vi "TektronixMDO_multiChannelReadout_writeFile.vi"(11 "file path":path=path "C:/Users/user01/Desktop/hsinyeh/SNSPD_Data/20230411/2.5M_6.1K_20photons_1.36uW_100mV") -> ()   [LabVIEW 2016]
doc: "This example illustrates how to use autosetup and continuously acquires waveforms from a single channel using the following steps:\n\n1. Specify a valid VISA session. \n2. Specify a channel. \n3. Specify a time-out value for reading waveform.\n4. Run the VI. The graph displays the waveform you acquire."
uses:
  <instrlib>/Tektronix DPO MSO 2000 4000 Series/Public/Configure/Configure Trigger (Edge).vi
  <instrlib>/Tektronix DPO MSO 2000 4000 Series/Public/Data/Read (Multiple Waveforms).vi
  <instrlib>/Tektronix DPO MSO 2000 4000 Series/Tektronix DPO MSO 2000 4000 Series.lvlib
panel:
  out "sum of values":dynamicdata(graph)=[{"t0"=timestamp(0.005 s since 1904-01-01), "dt"=0.01, "Y"=[0.0, 0.0, 0.0, 0.0, 0.0, 0.0, 0.0, 0.0, 0.0, 0.0, 0.0, 0.0, 0.0, 0.0, 0.0, 0.0, 0.0, 0.0, 0.0, 0.0, 0.0, 0.0, 0.0, 0.0, 0.0, 0.0, 0.0, 0.0, 0.0, 0.0, 0.0, 0.0, 0.0, 0.0, 0.0, 0.0, 0.0, 0.0, 0.0, 0.0, 0.0, 0.0, 0.0, 0.0, 0.0, 0.0, 0.0, 0.0, 0.0, 0.0], "attributes"=variant("NI_ChannelName"=variant(string "Summation (Histogram)"), "NI_ExpIsRelativeTime"=variant(bool TRUE), "NI_ExpStartTimeStamp"=variant(timestamp timestamp(0 s since 1904-01-01)), "NI_ExpTimeStamp"=variant(timestamp timestamp(0 s since 1904-01-01)), "NI_ExpXDimension"=variant(string "BIN"), "NI_OriginalChannelName"=variant(string "Summation"))}] caption="Histogram"
  in  "Enable Channel 3":bool
  in  "Vertical Coupling (1: DC) 3":u16(ring)=1 items=["AC", "DC", "Ground", "DC Reject"]
  in  "Probe Attenuation (1) 3":dbl=1.0
  in  "Vertical Offset (0.0 V) 3":dbl
  in  "Input Impedance 3":u16(ring) items=["1M", "75", "50"]
  in  "Vertical Range (10.0 V) 3":dbl=10.0
  in  "Bandwidth (0: FULL) 3":u16(ring) items=["FULL", "250 MHz", "150 MHz", "20 MHz"]
  in  "Enable Channel 4":bool
  in  "Input Impedance 4":u16(ring) items=["1M", "75", "50"]
  in  "Vertical Coupling (1: DC) 4":u16(ring)=1 items=["AC", "DC", "Ground", "DC Reject"]
  in  "Probe Attenuation (1) 4":dbl=1.0
  in  "Vertical Range (10.0 V) 4":dbl=10.0
  in  "Vertical Offset (0.0 V) 4":dbl
  in  "Bandwidth (0: FULL) 4":u16(ring) items=["FULL", "250 MHz", "150 MHz", "20 MHz"]
  in  "Enable Channel 2":bool=TRUE
  in  "Input Impedance 2":u16(ring)=2 items=["1M", "75", "50"]
  in  "Vertical Coupling (1: DC) 2":u16(ring)=1 items=["AC", "DC", "Ground", "DC Reject"]
  in  "Probe Attenuation (1) 2":dbl=1.0
  in  "Vertical Range (10.0 V) 2":dbl=1.0
  in  "Vertical Offset (0.0 V) 2":dbl
  in  "Bandwidth (0: FULL) 2":u16(ring) items=["FULL", "250 MHz", "150 MHz", "20 MHz"]
  in  "Input Impedance":u16(ring)=2 items=["1M", "75", "50"]
  in  "Vertical Coupling (1: DC)":u16(ring)=1 items=["AC", "DC", "Ground", "DC Reject"]
  in  "Vertical Range (10.0 V)":dbl=0.01
  in  "Vertical Offset (0.0 V)":dbl
  in  "Bandwidth (0: FULL)":u16(ring) items=["FULL", "250 MHz", "150 MHz", "20 MHz"]
  in  "Probe Attenuation (1)":dbl=1.0
  in  "Enable Channel":bool=TRUE
  in  "Trigger Source":u16(ring)=1 items=["Channel 1", "Channel 2", "Channel 3", "Channel 4", "AC Line", "Aux", "Digital Channel 0", "Digital Channel 1", "Digital Channel 2", "Digital Channel 3", "Digital Channel 4", "Digital Channel 5", "Digital Channel 6", "Digital Channel 7", "Digital Channel 8", "Digital Channel 9", "Digital Channel 10", "Digital Channel 11", "Digital Channel 12", "Digital Channel 13", "Digital Channel 14", "Digital Channel 15", "RF"]
  out "Event rate":dbl=1.5321756894790601
  in  "Maximum Time (10000ms)":u32=10000
  in  "Timebase (0.0005 s)":dbl=1e-08
  in  "Position (10 %)":dbl=10.0
  in  "Record Length":u32(ring)=10 items=["1000 points"=1, "10k points"=10, "100k points"=100, "1M points"=1000, "5M points"=5000, "10M points"=10000]
  out "Event Count":i32=75
  in  "Target total event":i32=1
  out "dt":dbl=4e-10 format="%#_13g"
  out "range":dynamicdata(graph)=[{"t0"=timestamp(0.00014999999999999996 s since 1904-01-01), "dt"=0.0003, "Y"=[0.0, 0.0, 0.0, 0.0, 0.0, 0.0, 0.0, 0.0, 0.0, 0.0, 0.0, 0.0, 0.0, 0.0, 0.0, 0.0, 0.0, 0.0, 0.0, 0.0, 0.0, 0.0, 0.0, 0.0, 0.0, 0.0, 0.0, 0.0, 0.0, 0.0, 0.0, 0.0, 0.0, 0.0, 0.0, 0.0, 0.0, 0.0, 0.0, 0.0, 0.0, 0.0, 0.0, 0.0, 0.0, 0.0, 0.0, 0.0, 0.0, 0.0, 0.0, 0.0, 0.0, 0.0, 0.0, 0.0, 0.0, 0.0, 0.0, 0.0, 0.0, 0.0, 0.0, 0.0, 0.0, 0.0, 0.0, 0.0, 0.0, 0.0, 0.0, 0.0, 0.0, 0.0, 0.0, 0.0, 0.0, 0.0, 0.0, 0.0, 0.0, 0.0, 0.0, 0.0, 0.0, 0.0, 0.0, 0.0, 0.0, 0.0, 0.0, 0.0, 0.0, 0.0, 0.0, 0.0, 0.0, 0.0, 0.0, 0.0], "attributes"=variant("NI_ChannelName"=variant(string "Range (Histogram)"), "NI_ExpIsRelativeTime"=variant(bool TRUE), "NI_ExpStartTimeStamp"=variant(timestamp timestamp(0 s since 1904-01-01)), "NI_ExpTimeStamp"=variant(timestamp timestamp(0 s since 1904-01-01)), "NI_ExpXDimension"=variant(string "BIN"), "NI_OriginalChannelName"=variant(string "Range"))}] caption="Histogram"
  in  "Operator":string="Hsin-Yeh"
  in  "Trigger Slope (0: Rising)":u16(ring)=1 items=["Rising", "Falling", "Either"]
  in  "Trigger Level (0.0 V)":dbl=-0.5
  in  "Trigger Coupling (0 : DC)":u16(ring) items=["DC", "HF Reject", "LF Reject", "Noise Reject", "AC"]
  out "Waveform Graph":waveform(dbl)[](graph)=[{"t0"=timestamp(-1.916400000023799e-06 s since 1904-01-01), "dt"=4e-10, "Y"=array[10000 elements]}, {"t0"=timestamp(-1.916400000023799e-06 s since 1904-01-01), "dt"=4e-10, "Y"=array[10000 elements]}]
  in  "stop":bool
  in  "VISA Resource Name":refnum<visa-resource-name>="USB0::0x0699::0x0408::C022314::INSTR"
  # "Channel 4"
  # "Channel 3"
  # "Channel 2"
  # "Channel 1"
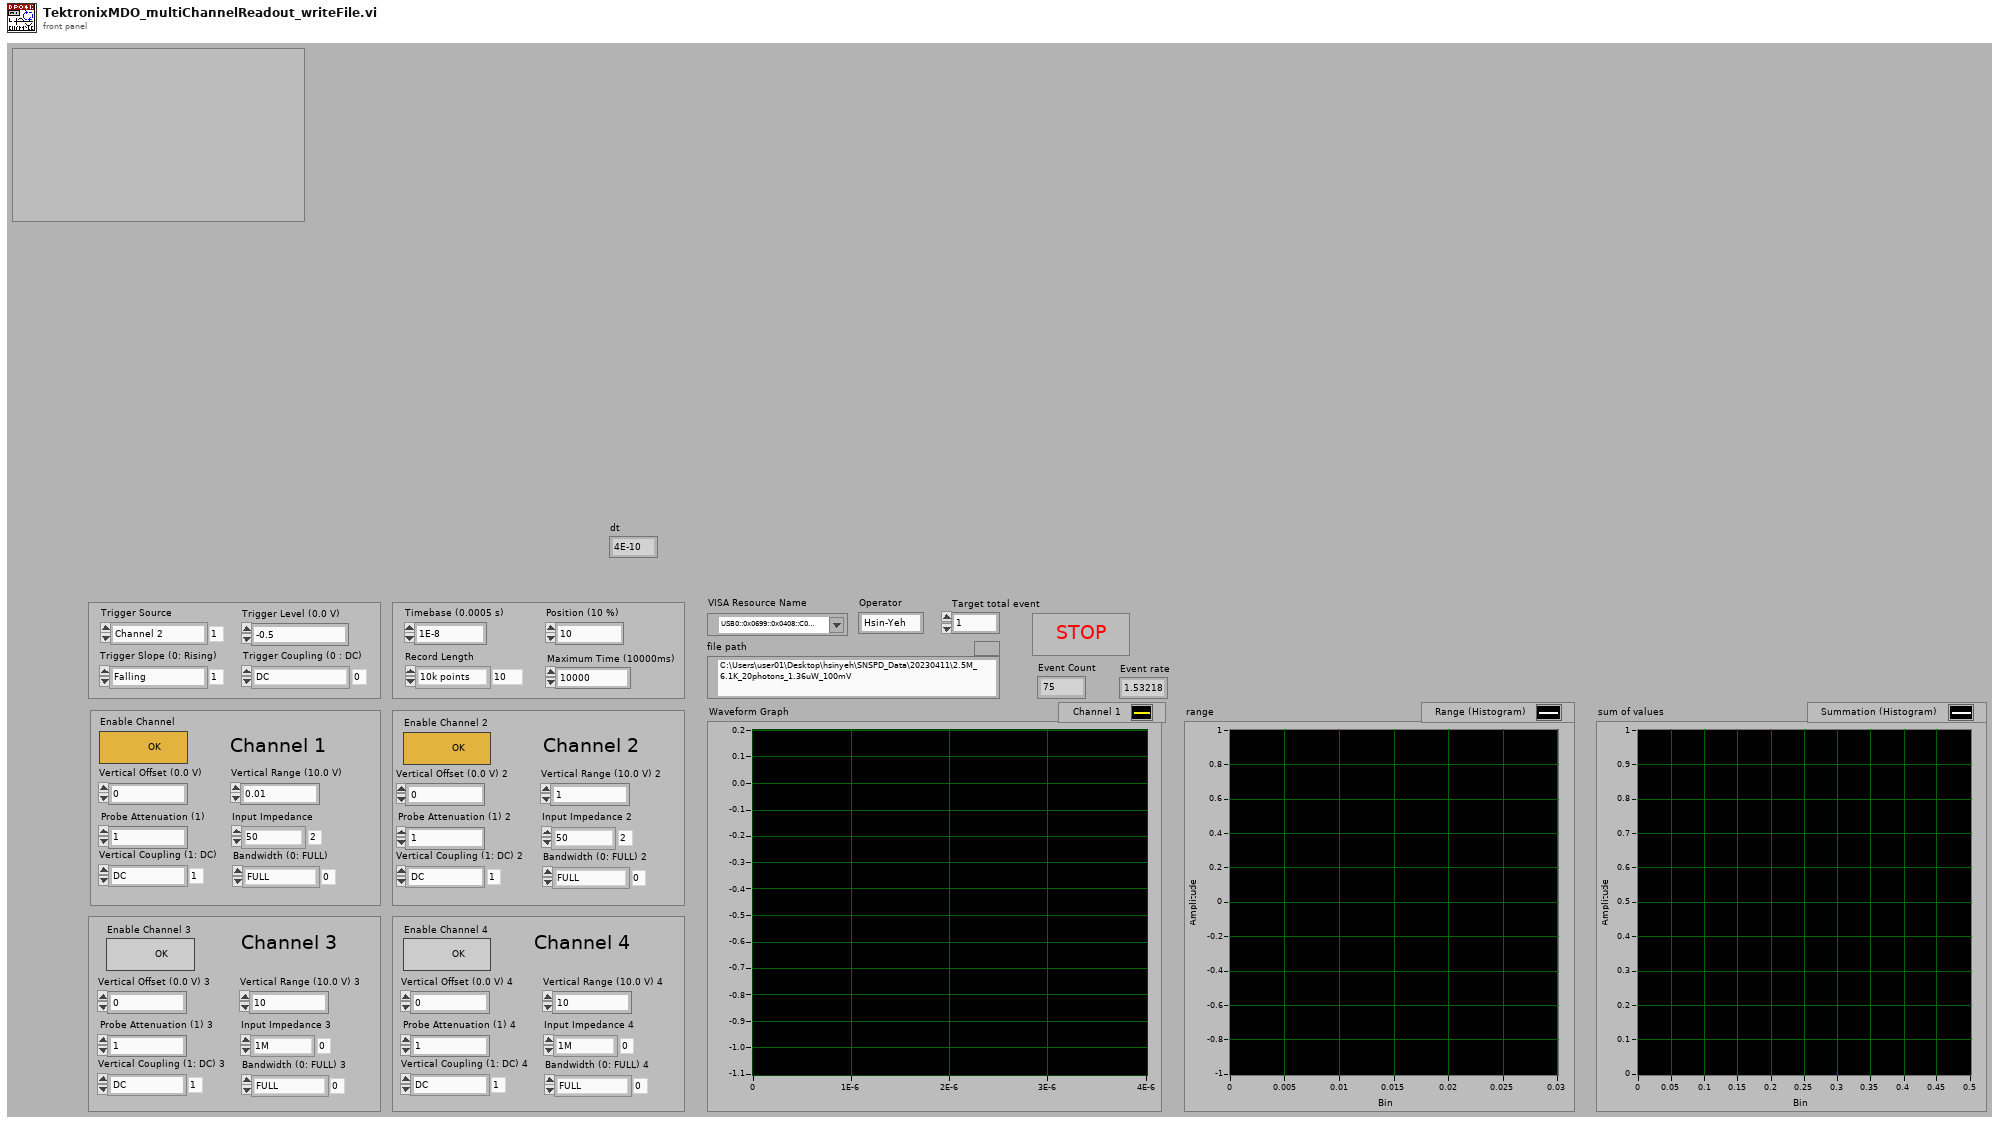
[diagram p1: front panel]
types:
  T1 = enum16{"open", "open or create", "create or replace", "create", "open (read-only)"}
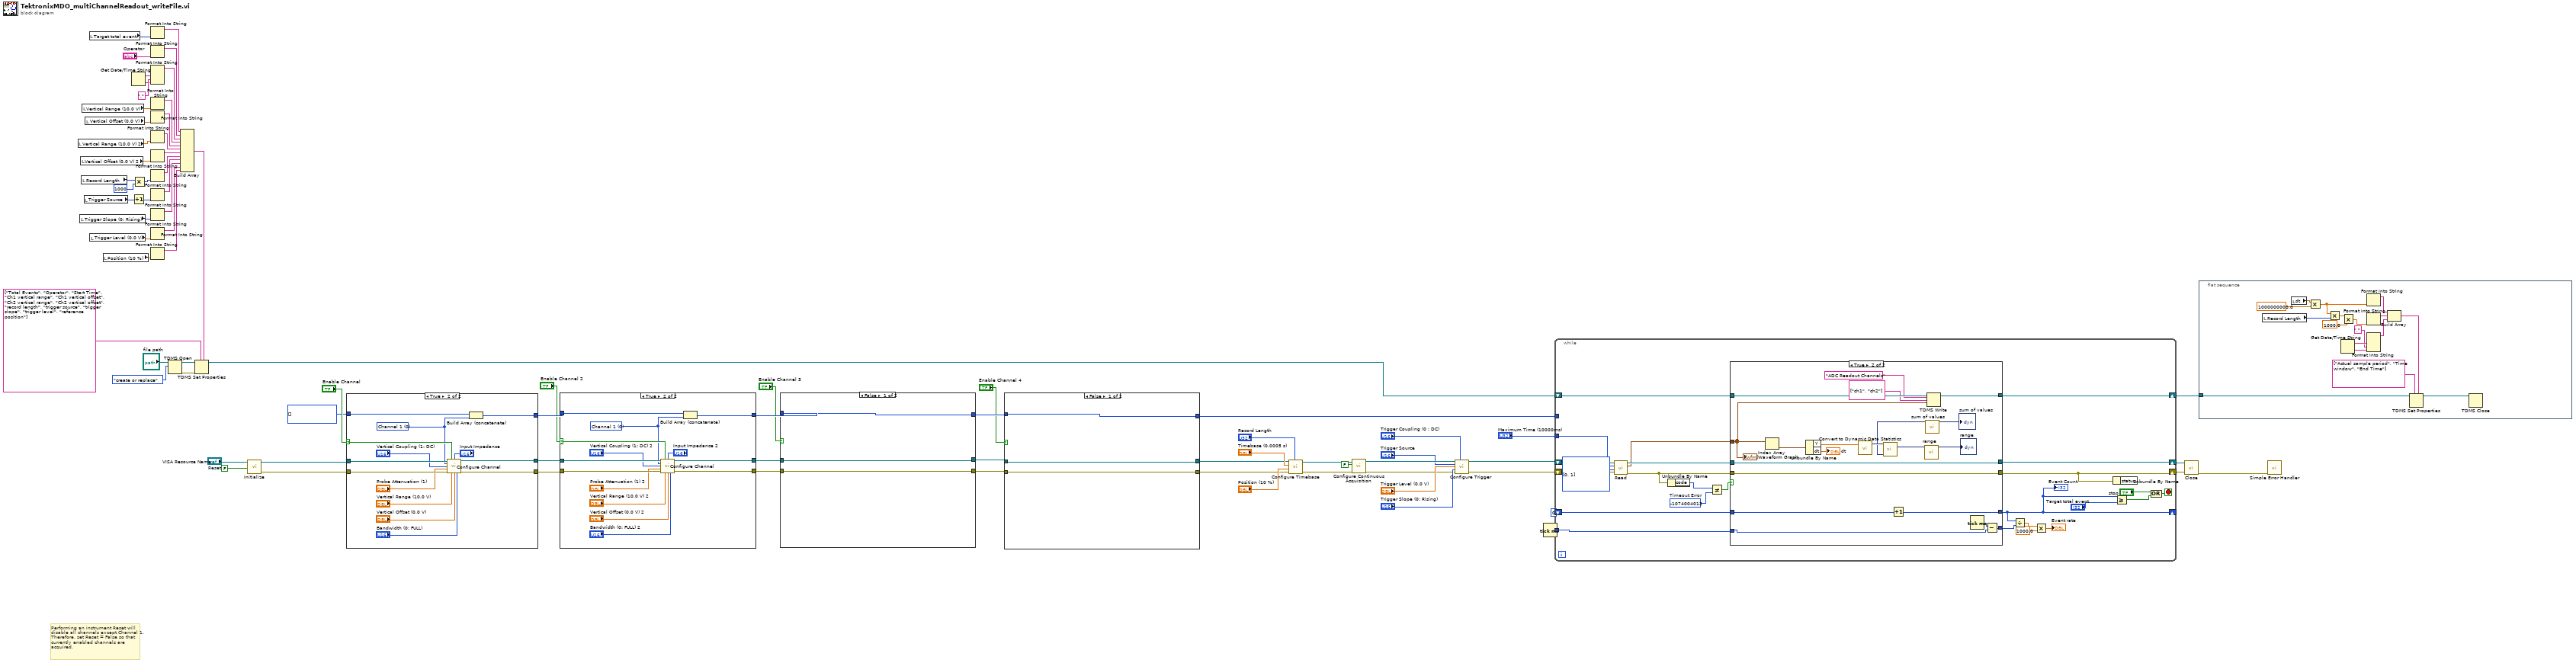
[diagram p0: block diagram]
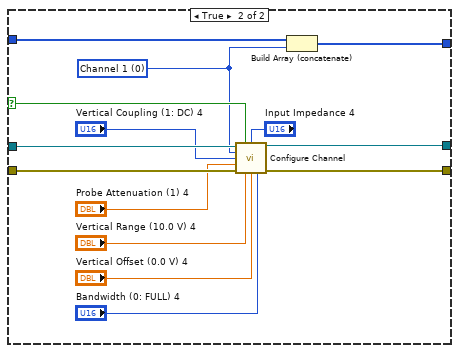
[diagram p2: hidden frame]
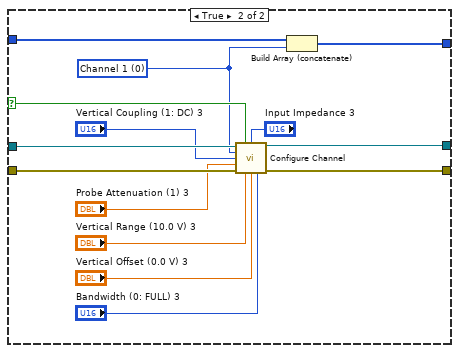
[diagram p3: hidden frame]
diagram:
  w27 = u16[] [] items=["Channel 1", "Channel 2", "Channel 3", "Channel 4", "Math", "Reference 1", "Reference 2", "Reference 3", "Reference 4", "Bus 1", "Bus 2"] ("Channel (0: Channel 1)")
  w75 = FALSE  # Reset
  # "Performing an instrument Reset will disable all channels except Channel 1. Therefore, set Reset = False so that currently enabled channels are acquired."
  n1 = local read "Vertical Range (10.0 V) 2"() -> (w6:dbl)
  n2 = local read "Trigger Slope (0: Rising)"() -> (w50:u16)
  n3 = local read "Vertical Offset (0.0 V) 2"() -> (w5:dbl)
  n4 = local read "Record Length"() -> (w8:u32)
  n5 = local read "Vertical Range (10.0 V)"() -> (w60:dbl)
  n6 = local read "Trigger Source"() -> (w3:u16)
  n7 = local read "Vertical Offset (0.0 V)"() -> (w58:dbl)
  n8 = local read "Target total event"() -> (w38:i32)
  n9 = local read "Trigger Level (0.0 V)"() -> (w61:dbl)
  n10 = local read "Position (10 %)"() -> (w59:dbl)
  n11 = Get Date/Time String() -> (date string=w56:string, time string=w54:string)  [unwired: 3 in]
  n12 = Increment(x=w3) -> (x+1=w2:u16)
  n13 = Multiply(x=w8, y=u32 1000) -> (x*y=w9:u32)
  n14 = Format Into String(w38) -> (resulting string=w62:string)  [unwired: 3 in, 1 out]
  n15 = Format Into String("Operator") -> (resulting string=w53:string)  [unwired: 3 in, 1 out]
  n16 = Format Into String(w56, "," ("input 2"), w54) -> (resulting string=w52:string)  [unwired: 3 in, 1 out]
  n17 = Format Into String(w60) -> (resulting string=w51:string)  [unwired: 3 in, 1 out]
  n18 = Format Into String(w58) -> (resulting string=w48:string)  [unwired: 3 in, 1 out]
  n19 = Format Into String(w6) -> (resulting string=w49:string)  [unwired: 3 in, 1 out]
  n20 = Format Into String(w5) -> (resulting string=w47:string)  [unwired: 3 in, 1 out]
  n21 = Format Into String(w9) -> (resulting string=w46:string)  [unwired: 3 in, 1 out]
  n22 = Format Into String(w2) -> (resulting string=w45:string)  [unwired: 3 in, 1 out]
  n23 = Format Into String(w50) -> (resulting string=w44:string)  [unwired: 3 in, 1 out]
  n24 = Format Into String(w61) -> (resulting string=w43:string)  [unwired: 3 in, 1 out]
  n25 = Format Into String(w59) -> (resulting string=w42:string)  [unwired: 3 in, 1 out]
  n26 = TDMS Open(10:T1."create or replace" ("operation (0:open)"), 11:"file path") -> (0:w64:errorcluster, 3:w63:refnum<k34>)  [unwired: 5 in]
  n27 = Build Array(w62, w53, w52, w51, w48, w49, w47, w46, w45, w44, w43, w42) -> (w41:string[])
  n28 = TDMS Set Properties(5:w41, 7:string[] ["Total Events", "Operator", "Start Time", "Ch1 vertical range", "Ch1 vertical offset", "Ch2 vertical range", "Ch2 vertical offset", "record length", "trigger source", "trigger slope", "trigger level", "reference position"], 8:w64, 11:w63) -> (3:w10:refnum<k34>)  [unwired: 2 in, 3 out]
  n29 = call <instrlib>:"Initialize.vi"("Reset (True)"=w75, "VISA resource name"="VISA Resource Name") -> ("error out"=w72:errorcluster, "VISA resource name out"=w73:refnum<visa-resource-name>)  [unwired: 8 in]
  n30 = case shown="True" "Enable Channel" {
    selector: "Enable Channel" -> [_ w85]
    tunnel: w73 -> [w81 w95]
    tunnel: w72 -> [w80 w94]
    tunnel: [w81 w87] -> w26
    tunnel: [w80 w86] -> w25
    tunnel: w27 -> [w79 w84]
    tunnel: [w79 w82] -> w18
    frame False {
    }
    frame True {
      w83 = u16 0 items=["Channel 1", "Channel 2", "Channel 3", "Channel 4", "Math", "Reference 1", "Reference 2", "Reference 3", "Reference 4", "Bus 1", "Bus 2"] ("Channel (0: Channel 1)")
      n31 = call <instrlib>:"Configure Channel.vi"("VISA resource name"=w95, "Enable Channel (T: Enable)"=w85, "Input Impedance (0: 1M ohm)"="Input Impedance", "Channel (0: Channel 1)"=w83, "Vertical Coupling (1: DC)"="Vertical Coupling (1: DC)", "Probe Attenuation (1)"="Probe Attenuation (1)", "error in (no error)"=w94, "Vertical Range (10.0 V)"="Vertical Range (10.0 V)", "Vertical Offset (0.0 V)"="Vertical Offset (0.0 V)", "Bandwidth (0: FULL)"="Bandwidth (0: FULL)") -> ("VISA resource name out"=w87:refnum<visa-resource-name>, "error out"=w86:errorcluster)  [unwired: 4 in]
      n32 = Build Array (concatenate)(w84, w83) -> (w82:u16[])
    }
  }
  n33 = case shown="True" "Enable Channel 2" {
    selector: "Enable Channel 2" -> [_ w102]
    tunnel: w26 -> [w98 w112]
    tunnel: w25 -> [w97 w111]
    tunnel: [w98 w104] -> w24
    tunnel: [w97 w103] -> w23
    tunnel: w18 -> [w96 w101]
    tunnel: [w96 w99] -> w17
    frame False {
    }
    frame True {
      w100 = u16 0 items=["Channel 1", "Channel 2", "Channel 3", "Channel 4", "Math", "Reference 1", "Reference 2", "Reference 3", "Reference 4", "Bus 1", "Bus 2"] ("Channel (0: Channel 1)")
      n34 = call <instrlib>:"Configure Channel.vi"("VISA resource name"=w112, "Enable Channel (T: Enable)"=w102, "Input Impedance (0: 1M ohm)"="Input Impedance 2", "Channel (0: Channel 1)"=w100, "Vertical Coupling (1: DC)"="Vertical Coupling (1: DC) 2", "Probe Attenuation (1)"="Probe Attenuation (1) 2", "error in (no error)"=w111, "Vertical Range (10.0 V)"="Vertical Range (10.0 V) 2", "Vertical Offset (0.0 V)"="Vertical Offset (0.0 V) 2", "Bandwidth (0: FULL)"="Bandwidth (0: FULL) 2") -> ("VISA resource name out"=w104:refnum<visa-resource-name>, "error out"=w103:errorcluster)  [unwired: 4 in]
      n35 = Build Array (concatenate)(w101, w100) -> (w99:u16[])
    }
  }
  n36 = case shown="False" "Enable Channel 3" {
    selector: "Enable Channel 3" -> [_ w119]
    tunnel: w24 -> [w115 w129]
    tunnel: w23 -> [w114 w128]
    tunnel: [w115 w121] -> w22
    tunnel: [w114 w120] -> w21
    tunnel: w17 -> [w113 w118]
    tunnel: [w113 w116] -> w16
    frame False {
    }
    frame True {
      w117 = u16 0 items=["Channel 1", "Channel 2", "Channel 3", "Channel 4", "Math", "Reference 1", "Reference 2", "Reference 3", "Reference 4", "Bus 1", "Bus 2"] ("Channel (0: Channel 1)")
      n37 = call <instrlib>:"Configure Channel.vi"("VISA resource name"=w129, "Enable Channel (T: Enable)"=w119, "Input Impedance (0: 1M ohm)"="Input Impedance 3", "Channel (0: Channel 1)"=w117, "Vertical Coupling (1: DC)"="Vertical Coupling (1: DC) 3", "Probe Attenuation (1)"="Probe Attenuation (1) 3", "error in (no error)"=w128, "Vertical Range (10.0 V)"="Vertical Range (10.0 V) 3", "Vertical Offset (0.0 V)"="Vertical Offset (0.0 V) 3", "Bandwidth (0: FULL)"="Bandwidth (0: FULL) 3") -> ("VISA resource name out"=w121:refnum<visa-resource-name>, "error out"=w120:errorcluster)  [unwired: 4 in]
      n38 = Build Array (concatenate)(w118, w117) -> (w116:u16[])
    }
  }
  n39 = case shown="False" "Enable Channel 4" {
    selector: "Enable Channel 4" -> [_ w136]
    tunnel: w22 -> [w132 w146]
    tunnel: w21 -> [w131 w145]
    tunnel: [w132 w138] -> w20
    tunnel: [w131 w137] -> w19
    tunnel: w16 -> [w130 w135]
    tunnel: [w130 w133] -> w11
    frame False {
    }
    frame True {
      w134 = u16 0 items=["Channel 1", "Channel 2", "Channel 3", "Channel 4", "Math", "Reference 1", "Reference 2", "Reference 3", "Reference 4", "Bus 1", "Bus 2"] ("Channel (0: Channel 1)")
      n40 = call <instrlib>:"Configure Channel.vi"("VISA resource name"=w146, "Enable Channel (T: Enable)"=w136, "Input Impedance (0: 1M ohm)"="Input Impedance 4", "Channel (0: Channel 1)"=w134, "Vertical Coupling (1: DC)"="Vertical Coupling (1: DC) 4", "Probe Attenuation (1)"="Probe Attenuation (1) 4", "error in (no error)"=w145, "Vertical Range (10.0 V)"="Vertical Range (10.0 V) 4", "Vertical Offset (0.0 V)"="Vertical Offset (0.0 V) 4", "Bandwidth (0: FULL)"="Bandwidth (0: FULL) 4") -> ("VISA resource name out"=w138:refnum<visa-resource-name>, "error out"=w137:errorcluster)  [unwired: 4 in]
      n41 = Build Array (concatenate)(w135, w134) -> (w133:u16[])
    }
  }
  n42 = call <instrlib>:"Configure Timebase.vi"("Record Length (10: 10k points)"="Record Length", "error in (no error)"=w19, "Position (10 %)"="Position (10 %)", "Timebase (0.0005 s)"="Timebase (0.0005 s)", "VISA resource name"=w20) -> ("error out"=w32:errorcluster, "VISA resource name out"=w34:refnum<visa-resource-name>)  [unwired: 5 in]
  n43 = call <instrlib>:"Configure Continuous Acquisition.vi"("error in (no error)"=w32, "Enable Continuous Acquisition Mode (T: Enable)"=FALSE, "VISA resource name"=w34) -> ("error out"=w31:errorcluster, "VISA resource name out"=w33:refnum<visa-resource-name>)  [unwired: 7 in]
  n44 = call-poly <instrlib>:"Configure Trigger.vi"("VISA resource name"=w33, "Trigger Coupling (0 : DC)"="Trigger Coupling (0 : DC)", "Trigger Source (0: Channel 1)"="Trigger Source", "Trigger Level (0.0 V)"="Trigger Level (0.0 V)", "Trigger Slope (0: Rising)"="Trigger Slope (0: Rising)", "error in (no error)"=w31) -> ("VISA resource name out"=w40:refnum<visa-resource-name>, "error out"=w36:errorcluster)  [unwired: 8 in]
  n45 = Tick Count (ms)() -> (millisecond timer value=w29:u32)
  n46 = while {
    tunnel: "Maximum Time (10000ms)" -> [w170]
    shift-right: [w167] -> w77
    shift-left: w40 -> [w169]
    shift-right: [w157] -> w4
    shift-left: w10 -> [w158]
    shift-right: [w153] -> _
    shift-left: 0 -> [w163]
    shift-right: [w155] -> w35
    shift-left: w36 -> [w156]
    tunnel: w29 -> [w154]
    tunnel: w11 -> [_]
    stop <- w159 stop-if-true
    w147 = u16[] [0, 1] items=["Channel 1", "Channel 2", "Channel 3", "Channel 4", "Math", "Reference 1", "Reference 2", "Reference 3", "Reference 4", "D0", "D1", "D2", "D3", "D4", "D5", "D6", "D7", "D8", "D9", "D10", "D11", "D12", "D13", "D14", "D15", "Amplitude", "Frequency", "Phase", "Normal", "Average", "Maximum Peak Hold", "Minimum Peak Hold"] ("Channels")
    w165 = -1074004013  # Timeout Error
    n47 = call-poly <instrlib>:"Read.vi"("error in (no error)"=w156, "Maximum Time (10000ms)"=w170, "Channels"=w147, "VISA resource name"=w169) -> ("error out"=w155:errorcluster, "Waveform Data"=w148:waveform(dbl)[], "VISA resource name out"=w168:refnum<visa-resource-name>)  [unwired: 5 in]
    n48 = Unbundle By Name(w155) -> ("code"=w166:i32)
    n49 = Not Equal?(x=w166, y=w165) -> (x != y?=w164:bool)
    n50 = case shown="True" w164 {
      tunnel: w168 -> [w175 w189]
      tunnel: [w175 w189] -> w167
      tunnel: w155 -> [w174 w187]
      tunnel: [w174 w187] -> _
      tunnel: w163 -> [w173 w194]
      tunnel: [w173 w193] -> w153
      tunnel: w158 -> [w172 w192]
      tunnel: [w172 w190] -> w157
      tunnel: w148 -> [_ w179]
      tunnel: w154 -> [w171 w184]
      tunnel: [w171 w183] -> w152
      frame False {
      }
      frame True {
        n51 = Index Array(array=w179) -> (element=w182:waveform(dbl))  [unwired: 1 in]
        n52 = Unbundle By Name(w182) -> ("Y"=w181:dbl[], "dt"=→"dt":dbl)
        n53 = call "Convert to Dynamic Data"("Array"=w181) -> ("Dynamic Data Type"=w188:dynamicdata)  [unwired: 3 in]
        n54 = call "Statistics"("Signals"=w188) -> ("Summation"=w177:dynamicdata, "Range"=w186:dynamicdata)  [unwired: 24 in, 1 out]
        n55 = Increment(x=w194) -> (x+1=w193:i32)
        n56 = call "range"("Signal"=w186) -> ("Histogram"=→"range":dynamicdata)  [unwired: 9 in, 1 out]
        n57 = call "sum of values"("Signal"=w177) -> ("Histogram"=→"sum of values":dynamicdata)  [unwired: 9 in, 1 out]
        n58 = TDMS Write(0:w192, 5:"ADC Readout Channels" ("group name (Untitled)"), 7:string[] ["ch1", "ch2"], 9:w179) -> (4:w190:refnum<k34>)  [unwired: 2 in, 3 out]
        n59 = Tick Count (ms)() -> (millisecond timer value=w185:u32)
        n60 = Subtract(x=w185, y=w184) -> (x-y=w183:u32)
        "Waveform Graph" <- w179
      }
    }
    "Event Count" <- w153
    n61 = Divide(x=w153, y=w152) -> (x/y=w151:dbl)
    n62 = Multiply(x=w151, y=1000.0) -> (x*y=→"Event rate":dbl)
    n63 = Unbundle By Name(w155) -> ()  [unwired: 1 out]
    n64 = Greater Or Equal?(x=w153, y="Target total event") -> (x >= y?=w160:bool)
    n65 = Compound Arithmetic op=OR("stop", w160) -> (w159:bool)
  }
  n66 = call <instrlib>:"Close.vi"("error in (no error)"=w35, "VISA resource name"=w77) -> ("error out"=w76:errorcluster)  [unwired: 9 in]
  n67 = flat-sequence {
    tunnel: w4 -> [w208]
    frame #0 {
      n68 = local read "Record Length"() -> (w202:u32)
      n69 = local read "dt"() -> (w200:dbl)
      n70 = Multiply(x=w200, y=1000000000.0) -> (x*y=w199:dbl)
      n71 = Multiply(x=w199, y=w202) -> (x*y=w198:dbl)
      n72 = Get Date/Time String() -> (date string=w211:string, time string=w210:string)  [unwired: 3 in]
      n73 = Multiply(x=w198, y=1000.0) -> (x*y=w196:dbl)
      n74 = Format Into String(w199) -> (resulting string=w205:string)  [unwired: 3 in, 1 out]
      n75 = Format Into String(w196) -> (resulting string=w201:string)  [unwired: 3 in, 1 out]
      n76 = Format Into String(w211, "," ("input 2"), w210) -> (resulting string=w203:string)  [unwired: 3 in, 1 out]
      n77 = Build Array(w205, w201, w203) -> (w204:string[])
      n78 = TDMS Set Properties(5:w204, 7:string[] ["Actual sample period", "Time window", "End Time"], 11:w208) -> (3:w212:refnum<k34>)  [unwired: 3 in, 3 out]
      n79 = TDMS Close(11:w212) -> ()  [unwired: 1 in, 2 out]
    }
  }
  n80 = call <vilib>:"Simple Error Handler.vi"("error in (no error)"=w76) -> ()  [unwired: 4 in, 5 out]
